vi "PH_Switch_USB.panel.vi"(0 "object ref":refnum<vi>, 5 "error in (no error)":errorcluster) -> (19 "error out":errorcluster)   [LabVIEW 2014, in "PH_Switch_USB.lvlib"]
doc: "By this VI a hardware switch can be monitored and switched. \n\nThe indicators \"FALSE\", \"TRUE\" and \"SWITCH STATE\" show the value of the Beckhoff-Tag: blue indicates bad tag status reference problems, darkgreen false and lightgreen true. If everything is working fine, \"FALSE\" and \"SWITCH STATE\" should show the same value, while \"TRUE\" has the opposite value. The caption of the sensors for \"FALSE\" and \"TRUE\" are taken out of the database. In case of only one or no sensor these GUI elements are not shown at all.\n\nThe oval button switches. It should be in the same state as the \"SWITCH STATE\" indicator. \n\n\"Delete Instance\" disconnects and removes the instance from the PCS.\n\n\nLicense Agreement for this software:\n\nCopyright (C)\nGesellschaft für Schwerionenforschung, GSI\nPlanckstr. 1\n64291 Darmstadt\nGermany\n\nContact: D.Beck@gsi.de \n\nThis program is free software; you can redistribute it and/or modify it under the terms of the GNU General Public License as published by the Free Software Foundation; either version 2 of the license, or (at your option) any later version.\n\nThis program is distributed in the hope that it will be useful, but WITHOUT ANYW ARRANTY; without even the implied warranty of MERCHANTABILITY or FITNESS FOR A PARTICULAR PURPOSE. See the GNU General License for more details (http://www.gnu.org).\n\nGesellschaft für Schwerionenforschung, GSI\nPlanckstr. 1, 64291 Darmstadt, Germany\nFor all questions and ideas contact: M.Richter@gsi.de, H.Brand@gsi.de or D.Beck@gsi.de.\nLast update: 18-DEC-2002"
uses:
  PH_Switch_USB.lvlib
  PH_Basics/PH_StatusHandler/PH_StatusHandler.GUI element.ctl
  CS_Core/CSObj/CSObj.lvlib
  CS_Core/CSSystem/CSSystemLib/CSSystemLib.lvlib
  PH_Basics/PH_Common/PH_Common.lvlib
  PH_Basics/PH_Class/PH_Class.lvlib
  PH_Basics/PH_StatusHandler/PH_StatusHandler.lvlib
panel:
  out "Status":T1 caption="Enabling State"
  in  "Exit":bool
  in  "Delete":bool
  in  "Knob":bool
  out "SW STATE":u32(colorbox)
  out "FALSE":u32(colorbox)
  out "TRUE":u32(colorbox)
  # "PCS"
  # "3.40"
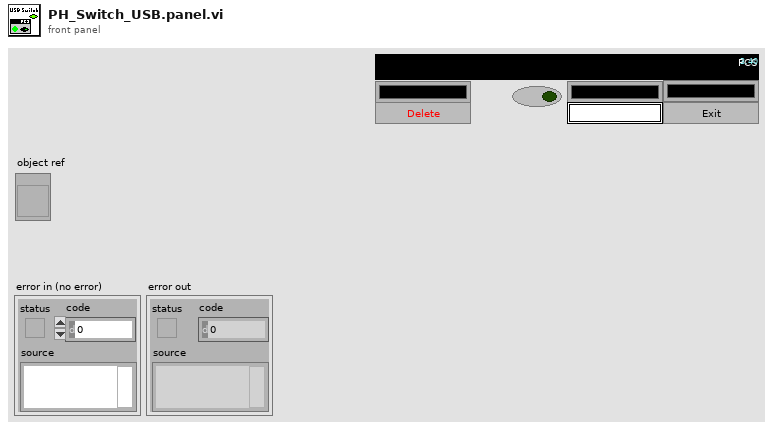
[diagram p1: front panel]
types:
  T1 = typedef "PH_StatusHandler.lvlib/PH_StatusHandler.GUI element.ctl" = u16
  T2 = typedef "PH_Switch_USB.lvlib/PH_Switch_USB.i attribute.ctl" = cluster{"GUI Refs":cluster{"GUI-Knob":refnum<vi>, "Delete":refnum<vi>}, "Switch":cluster{"GUI Ref":refnum<vi>, "Service name":string, "Array No.":i16, "caption":string, "Status":T3}, "True-Sensor":cluster{"GUI Ref":refnum<vi>, "Service name":string, "Array No.":i16, "caption":string, "Status":T3}, "False-Sensor":cluster{"GUI Ref":refnum<vi>, "Service name":string, "Array No.":i16, "caption":string, "Status":T3}}
  T3 = typedef "PH_StatusHandler.lvlib/PH_StatusHandler.Status.ctl" = i16
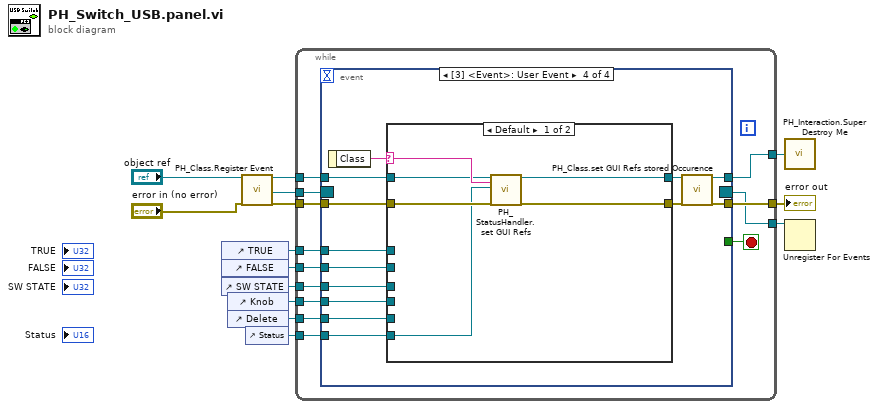
[diagram p0: block diagram]
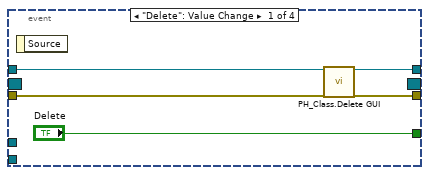
[diagram p2: hidden frame]
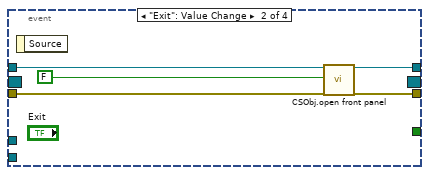
[diagram p3: hidden frame]
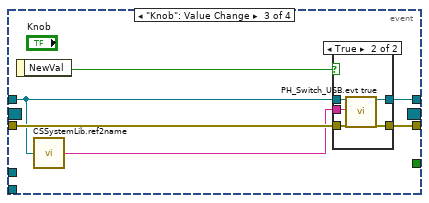
[diagram p4: hidden frame]
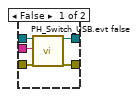
[diagram p5: hidden frame]
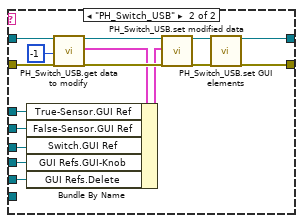
[diagram p6: hidden frame]
diagram:
  n1 = control-ref of="TRUE"() -> (w6:refnum<vi>)
  n2 = control-ref of="FALSE"() -> (w5:refnum<vi>)
  n3 = control-ref of="SW STATE"() -> (w4:refnum<vi>)
  n4 = control-ref of="Knob"() -> (w3:refnum<vi>)
  n5 = control-ref of="Delete"() -> (w2:refnum<vi>)
  n6 = call "PH_Class.Register Event.vi"("i ref in"="object ref", "error in (no error)"="error in (no error)") -> ("i ref out"=w12:refnum<vi>, "Event Registration Refnum"=w10:refnum<event-registration>, "error out"=w11:errorcluster)  [unwired: 15 in]
  n7 = control-ref of="Status"() -> (w1:refnum<vi>)
  n8 = while {
    tunnel: w12 -> [w24]
    tunnel: [w23] -> w14
    tunnel: w11 -> [w26]
    tunnel: [w25] -> w13
    tunnel: w10 -> [w22]
    tunnel: [w21] -> w9
    tunnel: w6 -> [w20]
    tunnel: w5 -> [w19]
    tunnel: w4 -> [w18]
    tunnel: w3 -> [w17]
    tunnel: w2 -> [w16]
    tunnel: w1 -> [w15]
    stop <- w27 stop-if-true
    n9 = event shown="[3] <Event>: User Event" {
      selector: w22 -> [_ _ _ _]
      dyn-events: [_ _ _ _] -> w21
      timeout: _ -> [_ _ _ _]
      tunnel: ["Delete" _ _ _] -> w27
      tunnel: w24 -> [w31 w36 w40 w64]
      tunnel: w26 -> [w30 w35 w43 w62]
      tunnel: [w29 w34 w42 w65] -> w25
      tunnel: [w28 w33 w38 w66] -> w23
      tunnel: w20 -> [_ _ _ w60]
      tunnel: w19 -> [_ _ _ w58]
      tunnel: w18 -> [_ _ _ w57]
      tunnel: w17 -> [_ _ _ w56]
      tunnel: w16 -> [_ _ _ w55]
      tunnel: w15 -> [_ _ _ w54]
      event "Delete": Value Change {
        n10 = event-data() -> ()  [unwired: 1 in, 1 out]
        n11 = call "PH_Class.Delete GUI.vi"("VI in"=w31, "error in (no error)"=w30) -> ("VI out"=w28:refnum<vi>, "error out"=w29:errorcluster)  [unwired: 16 in]
      }
      event "Exit": Value Change {
        n12 = event-data() -> ()  [unwired: 1 in, 1 out]
        n13 = call "CSObj.open front panel.vi"("i ref in"=w36, "frontPanelOpen"=FALSE ("front panel open"), "error in (no error)"=w35) -> ("i ref out"=w33:refnum<vi>, "error out"=w34:errorcluster)  [unwired: 15 in]
      }
      event "Knob": Value Change {
        n14 = event-data() -> ("NewVal"=w41:bool)  [unwired: 1 in]
        n15 = call "CSSystemLib.ref2name.vi"("obj refnum"=w40) -> ("name"=w39:string)
        n16 = case shown="True" w41 {
          tunnel: w40 -> [w48 w53]
          tunnel: w43 -> [w47 w52]
          tunnel: [w46 w51] -> w42
          tunnel: w39 -> [w45 w50]
          tunnel: [w44 w49] -> w38
          frame False {
            n17 = call "PH_Switch_USB.evt false.vi"("i ref in"=w48, "Instance"=w45, "error in (no error)"=w47) -> ("i ref out"=w44:refnum<vi>, "error out"=w46:errorcluster)  [unwired: 15 in]
          }
          frame True {
            n18 = call "PH_Switch_USB.evt true.vi"("i ref in"=w53, "Instance"=w50, "error in (no error)"=w52) -> ("i ref out"=w49:refnum<vi>, "error out"=w51:errorcluster)  [unwired: 15 in]
          }
        }
      }
      event User Event {
        n19 = event-data() -> ("Class"=w59:string)  [unwired: 1 in]
        n20 = case shown="Default" w59 {
          selector: w59 -> [w70 _]
          tunnel: w64 -> [w69 w83]
          tunnel: [w68 w74] -> w63
          tunnel: w62 -> [w72 w82]
          tunnel: [w71 w73] -> w61
          tunnel: w60 -> [_ w81]
          tunnel: w58 -> [_ w80]
          tunnel: w57 -> [_ w79]
          tunnel: w56 -> [_ w78]
          tunnel: w55 -> [_ w77]
          tunnel: w54 -> [w67 _]
          frame Default {
            n21 = call "PH_StatusHandler.set GUI Refs.vi"("i ref in"=w69, "Class"=w70, "GUI Ref"=w67, "error in (no error)"=w72) -> ("i ref out"=w68:refnum<vi>, "error out"=w71:errorcluster)  [unwired: 14 in]
          }
          frame "PH_Switch_USB" {
            n22 = call "PH_Switch_USB.get data to modify.vi"("i ref in"=w83, "ms timeout (10000)"=-1, "error in (no error)"=w82) -> ("i ref out"=w88:refnum<vi>, "i attribute"=w86:T2, "error out"=w87:errorcluster)  [unwired: 13 in, 1 out]
            n23 = Bundle By Name(cluster=w86, "True-Sensor.GUI Ref"=w81, "False-Sensor.GUI Ref"=w80, "Switch.GUI Ref"=w79, "GUI Refs.GUI-Knob"=w78, "GUI Refs.Delete"=w77) -> (w85:T2)
            n24 = call "PH_Switch_USB.set modified data.vi"("i ref in"=w88, "i attribute"=w85, "error in (no error)"=w87) -> ("i ref out"=w75:refnum<vi>, "error out"=w76:errorcluster)  [unwired: 15 in]
            n25 = call "PH_Switch_USB.set GUI elements.vi"("i ref in"=w75, "error in (no error)"=w76) -> ("i ref out"=w74:refnum<vi>, "error out"=w73:errorcluster)  [unwired: 16 in]
          }
        }
        n26 = call "PH_Class.set GUI Refs stored Occurence.vi"("i ref in"=w63, "error in (no error)"=w61) -> ("i ref out"=w66:refnum<vi>, "error out"=w65:errorcluster)  [unwired: 16 in]
      }
    }
  }
  "error out" <- w13
  n27 = call "PH_Interaction.Super Destroy Me.vi"("i ref out"=w14) -> ()
  n28 = Unregister For Events(event registration refnum=w9) -> ()  [unwired: 1 in, 1 out]
